vi "Read Defaults from INI File.vi"(8 "error in (no error)":errorcluster, 11 "Toggle 8 in":refnum<class "Toggle 8.lvclass">) -> (0 "error out":errorcluster, 3 "Toggle 8 out":refnum<class "Toggle 8.lvclass">)   [LabVIEW 2020, in "Toggle 8.lvclass"]
uses:
  Toggle 8.lvclass
  <vilib>/Utility/config.llb/Read Key (String).vi
  <vilib>/Utility/config.llb/NI_LVConfig.lvlib
  PIC-device/PIC-Device.lvclass
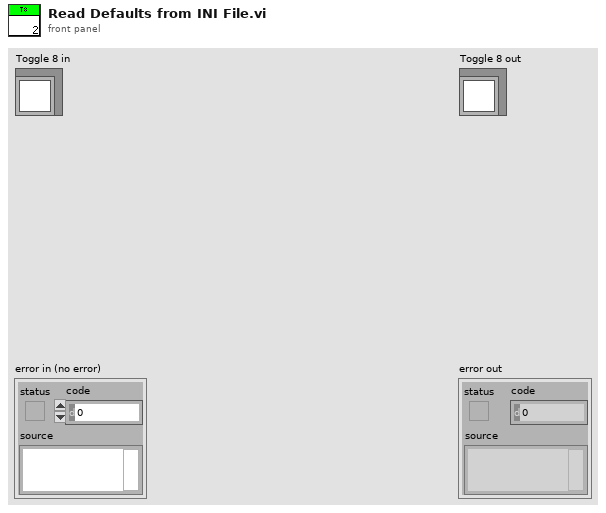
[diagram p1: front panel]
types:
  T1 = typedef "NI_LVConfig.lvlib/Config Data RefNum.ctl" = refnum<k1>
  T2 = typedef "Device.lvclass/Device Information Cluster.ctl" = cluster{"Device Info":string[][], "Default Values":T3[], "Fetched info":string[][]}
  T3 = typedef "PIC-Device.lvclass/Register to Write.ctl" = cluster{"Register":u32, "Value":u32, "Dev Address":u32, "Physical Adress":u32}
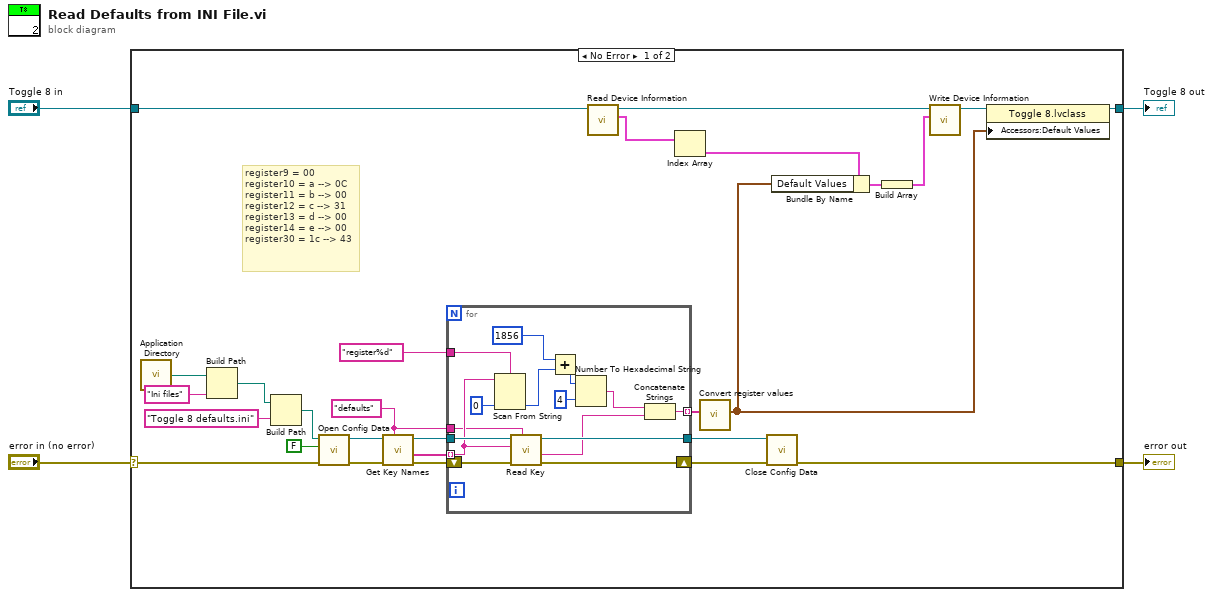
[diagram p0: block diagram]
diagram:
  n1 = case shown="No Error" "error in (no error)" {
    selector: "error in (no error)" -> [w17 w48]
    tunnel: [w16 w48] -> w3
    tunnel: [w13 w47] -> w1
    tunnel: "Toggle 8 in" -> [w12 w47]
    frame No Error {
      w21 = "defaults" ("section")
      # "register9 = 00\nregister10 = a --> 0C\nregister11 = b --> 00\nregister12 = c --> 31\nregister13 = d --> 00\nregister14 = e --> 00\nregister30 = 1c --> 43"
      n2 = call <vilib>:"Application Directory.vi"() -> ("Application Directory"=w31:path)
      n3 = Build Path(base path=w31, name or relative path="Ini files") -> (appended path=w18:path)
      n4 = Build Path(base path=w18, name or relative path="Toggle 8 defaults.ini") -> (appended path=w28:path)
      n5 = call <vilib>:"Open Config Data.vi"("error in (no error)"=w17, "create file if necessary (T)"=FALSE, "configuration file path"=w28) -> ("error out"=w26:errorcluster, "refnum"=w25:T1)  [unwired: 6 in, 1 out]
      n6 = call <vilib>:"Get Key Names.vi"("section"=w21, "error in (no error)"=w26, "refnum"=w25) -> ("error out"=w24:errorcluster, "key names"=w22:string[], "refnum out"=w23:T1)  [unwired: 5 in, 1 out]
      n7 = for {
        tunnel: w23 -> [w46]
        tunnel: w22 -> [w44] mode=indexing
        tunnel: w21 -> [w43]
        shift-right: [w42] -> w20
        shift-left: w24 -> [w45]
        tunnel: [w41] -> w19
        tunnel: [w38] -> w15 mode=indexing
        tunnel: "register%d" ("format string") -> [w37]
        n8 = Scan From String(format string=w37, input string=w44, default 1=u32 0) -> (output 1=w35:u32)  [unwired: 2 in, 3 out]
        n9 = call-poly <vilib>:"Read Key.vi"("section"=w43, "error in (no error)"=w45, "key"=w44, "refnum"=w46) -> ("error out"=w42:errorcluster, "value"=w39:string, "refnum out"=w41:T1)  [unwired: 4 in, 1 out]
        n10 = Add(x=u32 1856, y=w35) -> (x+y=w34:u32)
        n11 = Number To Hexadecimal String(1:i16 4 ("width (-)"), 2:w34) -> (0:w33:string)
        n12 = Concatenate Strings(w33, w39) -> (w38:string)
      }
      n13 = call-dynamic "Read Device Information.vi"("Device in"=w12) -> ("Device Info"=w9:T2[], "Device out"=w10:refnum<class "Toggle 8.lvclass">)  [unwired: 8 in, 1 out]
      n14 = Index Array(array=w9) -> (element=w8:T2)  [unwired: 1 in]
      n15 = call "Convert register values.vi"("Register strings"=w15) -> ("Register clusters out"=w7:T3[])  [unwired: 9 in, 1 out]
      n16 = call <vilib>:"Close Config Data.vi"("error in (no error)"=w20, "refnum"=w19) -> ("error out"=w16:errorcluster)  [unwired: 8 in, 1 out]
      n17 = Bundle By Name(cluster=w8, "Default Values"=w7) -> (w6:T2)
      n18 = Build Array(w6) -> (w5:T2[])
      n19 = call-dynamic "Write Device Information.vi"("Device Info"=w5, "Device in"=w10) -> ("Device out"=w11:refnum<class "Toggle 8.lvclass">)  [unwired: 8 in, 1 out]
      n20 = property class="Toggle 8.lvclass"(reference=w11, "Accessors:Default Values"=w7) -> (reference out=w13:refnum<class "Toggle 8.lvclass">)  [unwired: 1 in, 1 out]
    }
    frame Error {
    }
  }
  "error out" <- w3
  "Toggle 8 out" <- w1
